vi "Main.vi"() -> ()   [LabVIEW 2020]
uses:
  <vilib>/SAPHIR/ViBox - XControls/XTab/XTab.xctl
  Global.vi
panel:
  out "名称":string="C-EPS生产质量追溯系统"
  in  "XTab":refnum<vi>(xcontrol)
  out "时间：":string
  out "权限：":string
  out "用户：":string
  # "广东和氏工业技术集团股份有限公司"
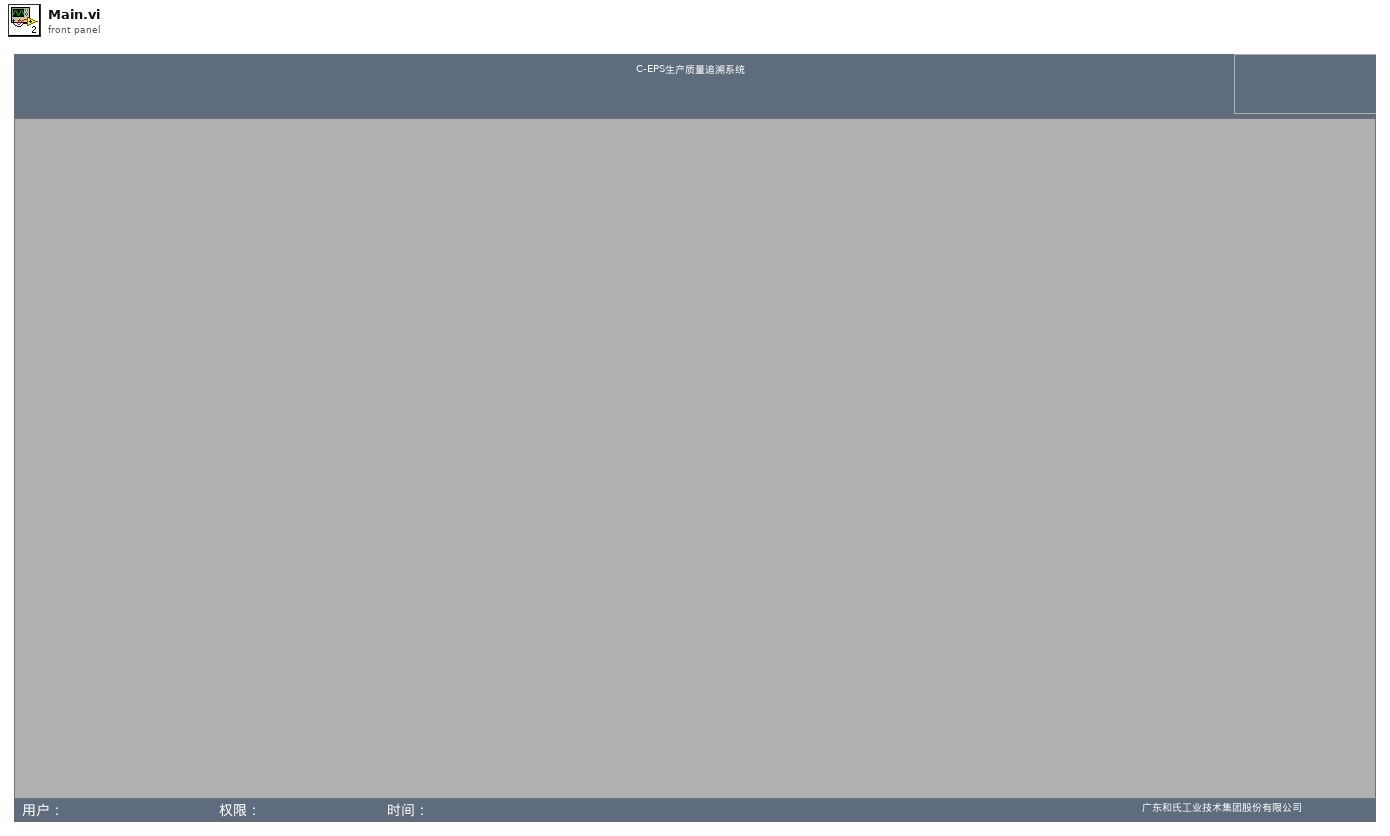
[diagram p1: front panel]
types:
  T1 = enum32{"Invalid", "Standard", "Closed", "Hidden", "Minimized", "Maximized"}
  T2 = cluster{"用户编号":string, "用户名":string, "用户密码(密文)":string, "用户权限":string}
  T3 = enum32{"invalid app kind", "Development System", "Run Time System", "Student Edition", "Embedded LabVIEW", "Evaluation", "Custom"}
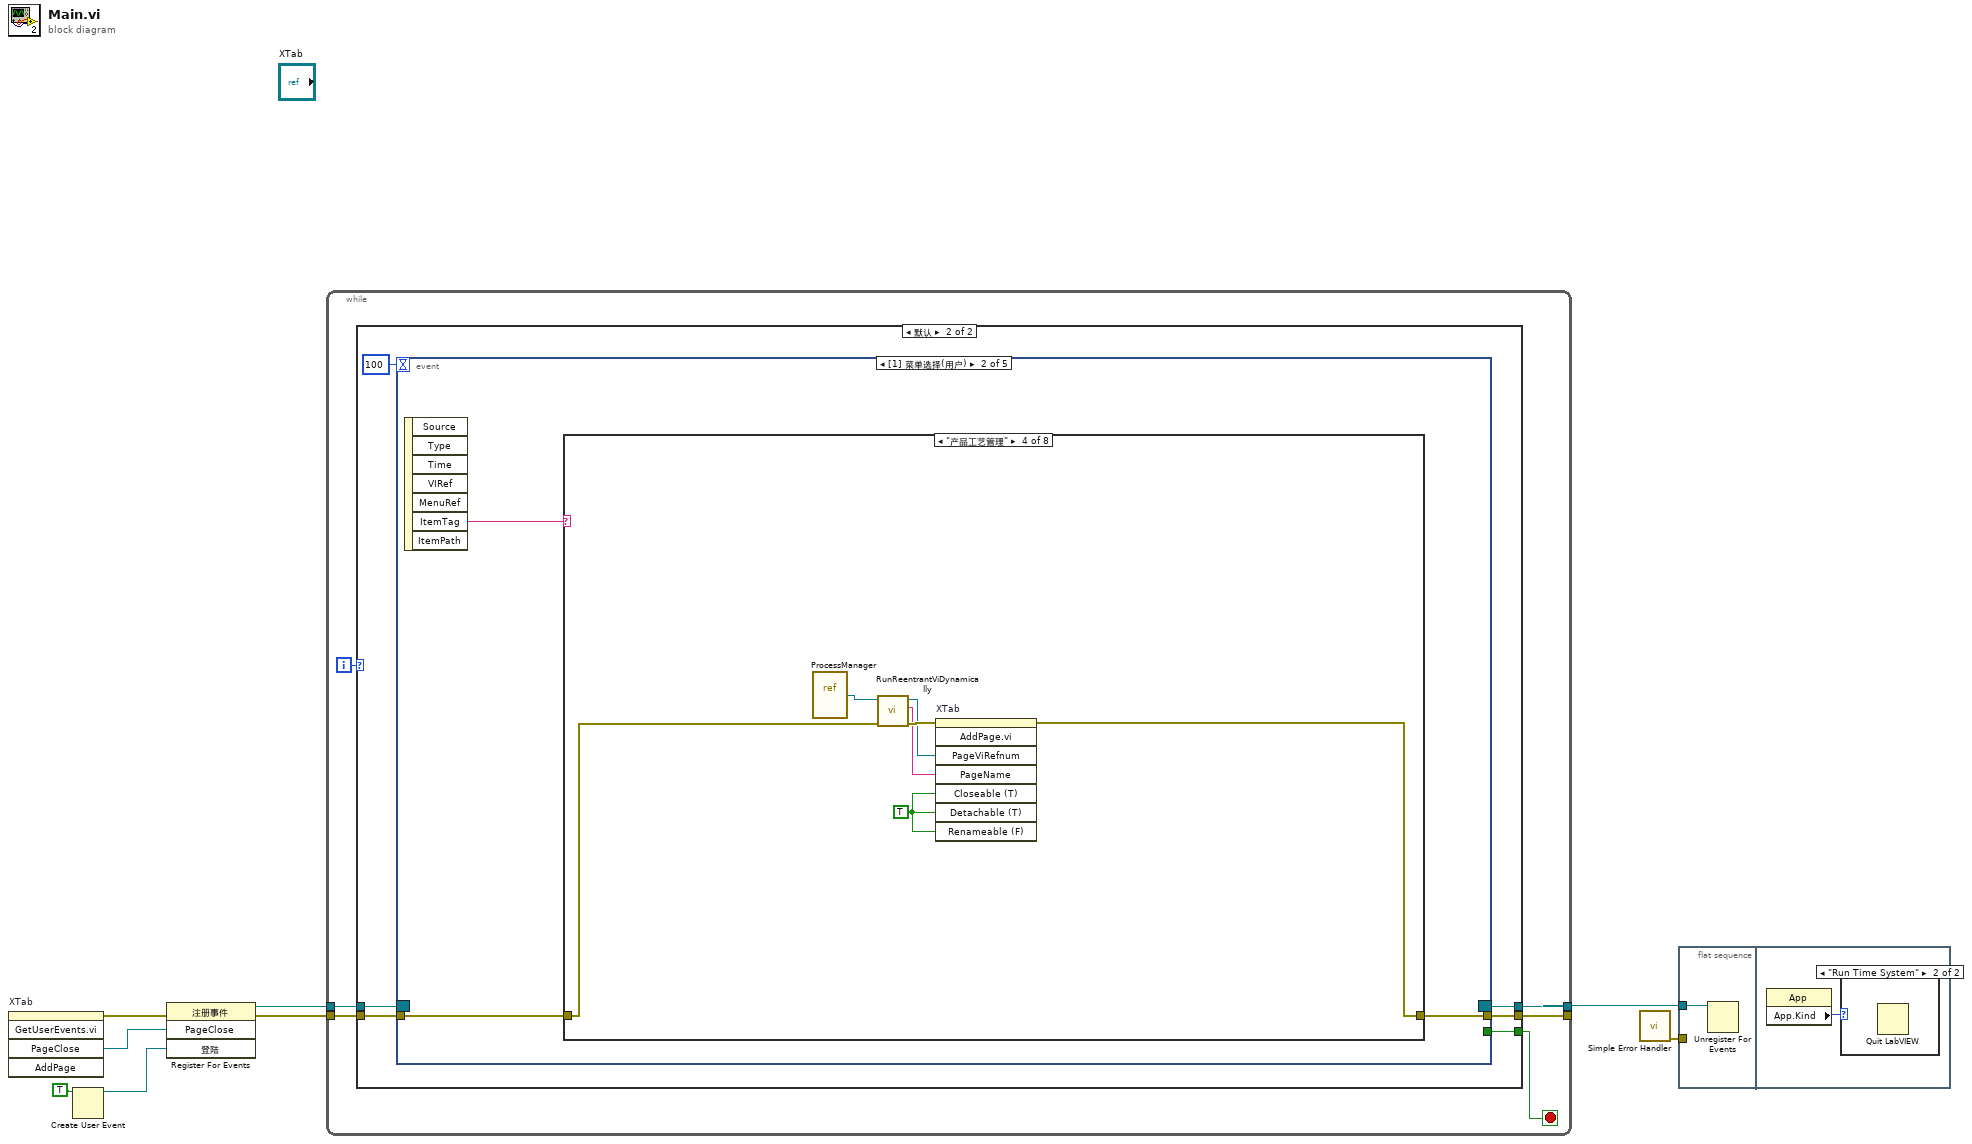
[diagram p0: block diagram]
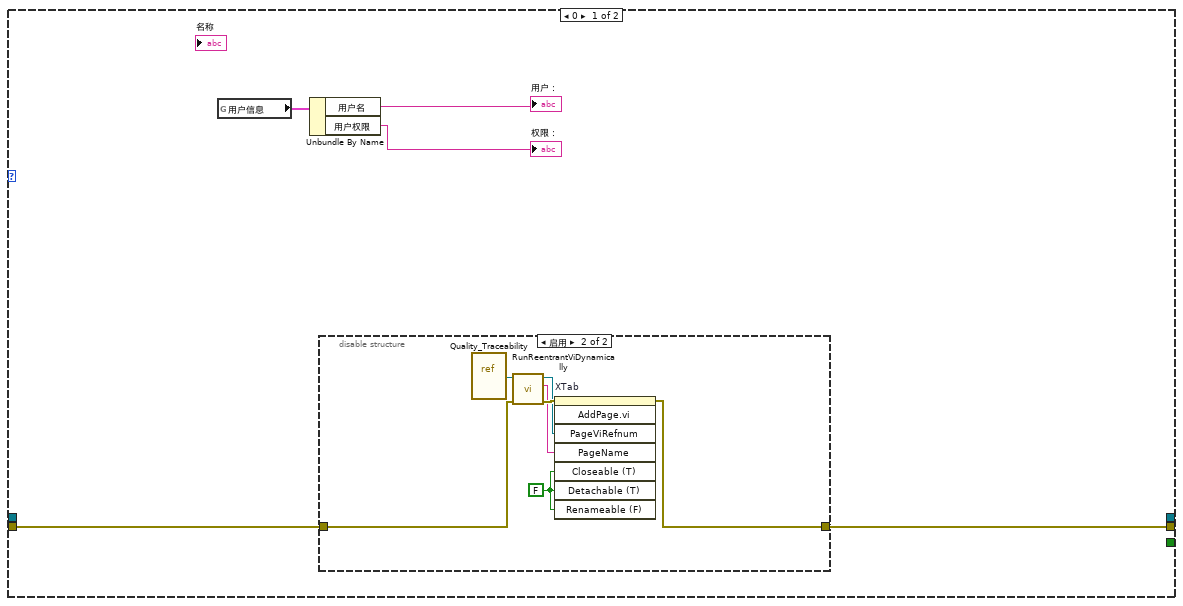
[diagram p3: hidden frame]
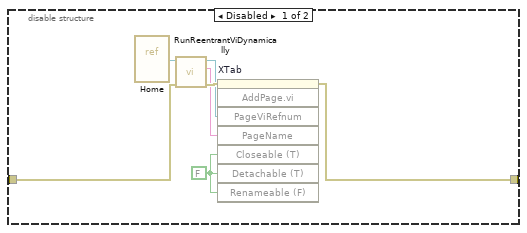
[diagram p4: hidden frame]
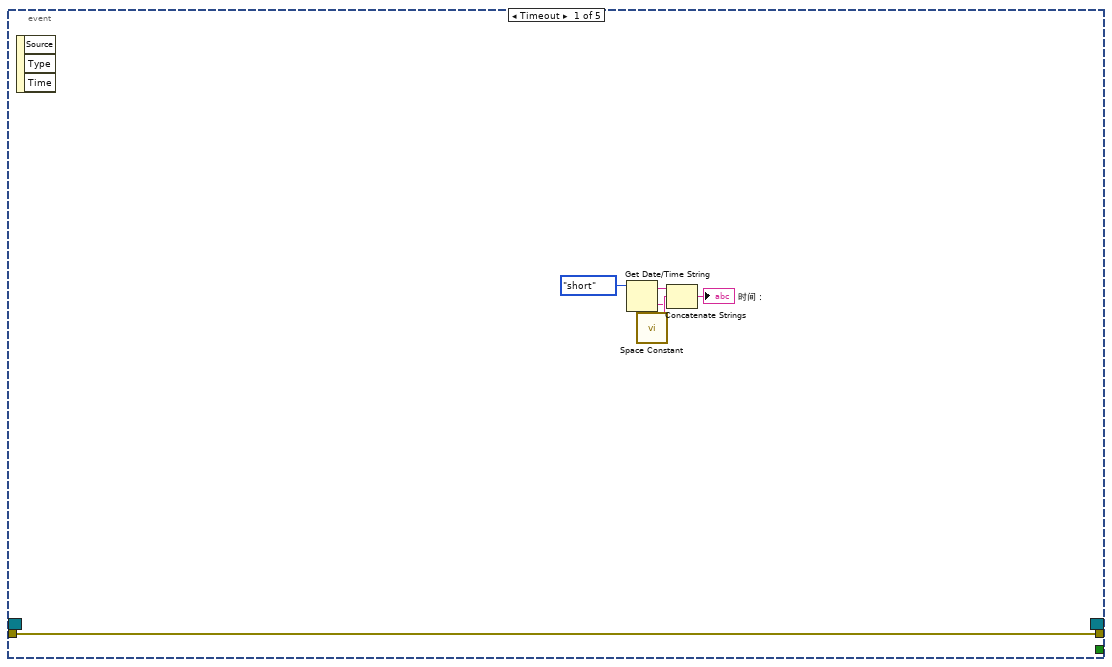
[diagram p5: hidden frame]
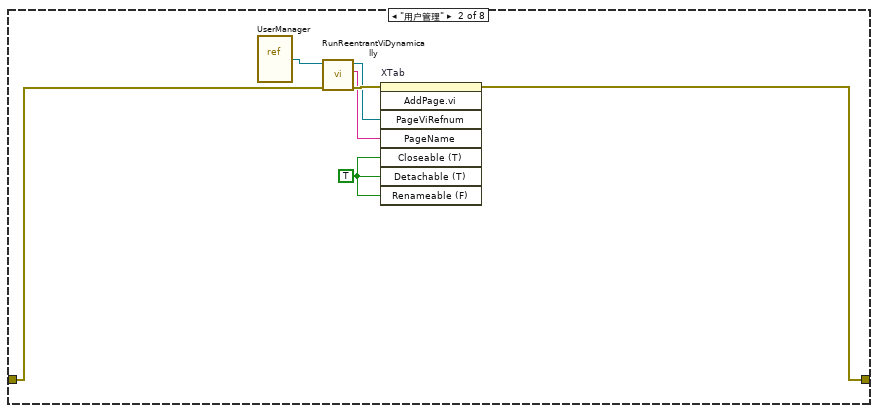
[diagram p7: hidden frame]
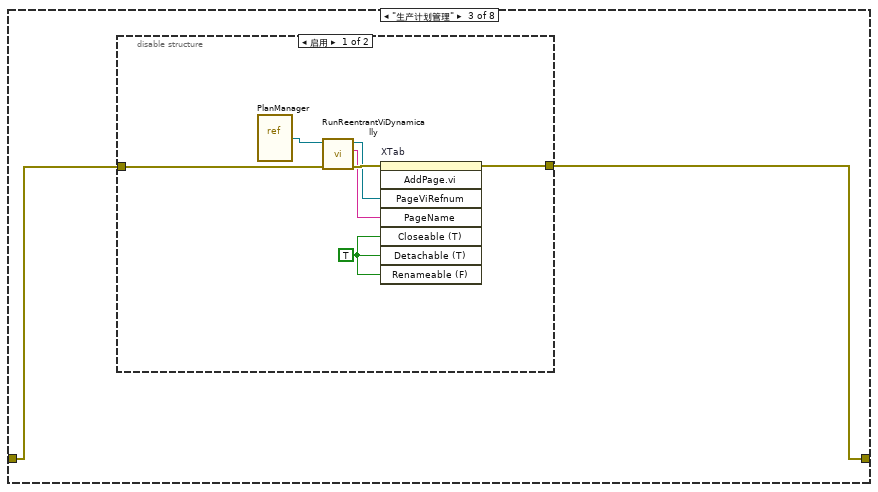
[diagram p8: hidden frame]
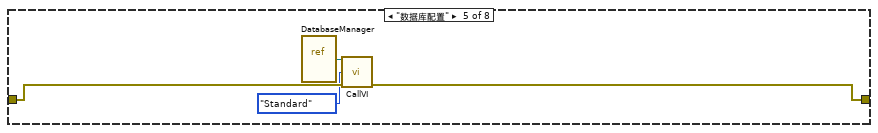
[diagram p10: hidden frame]
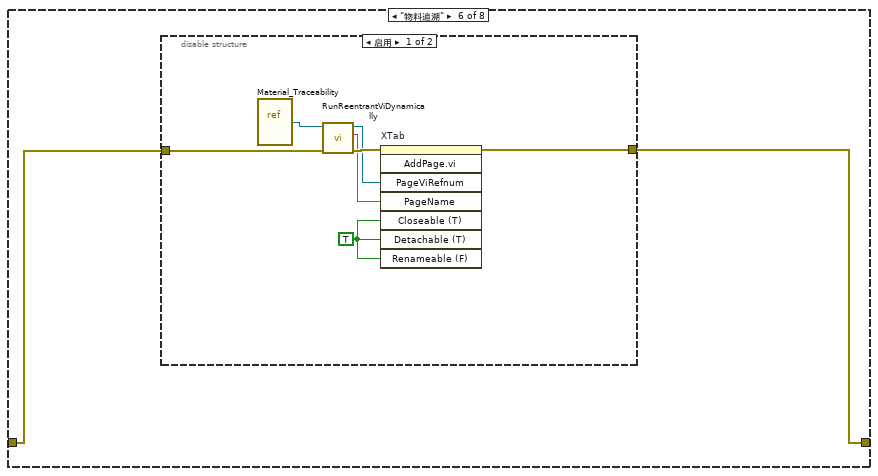
[diagram p11: hidden frame]
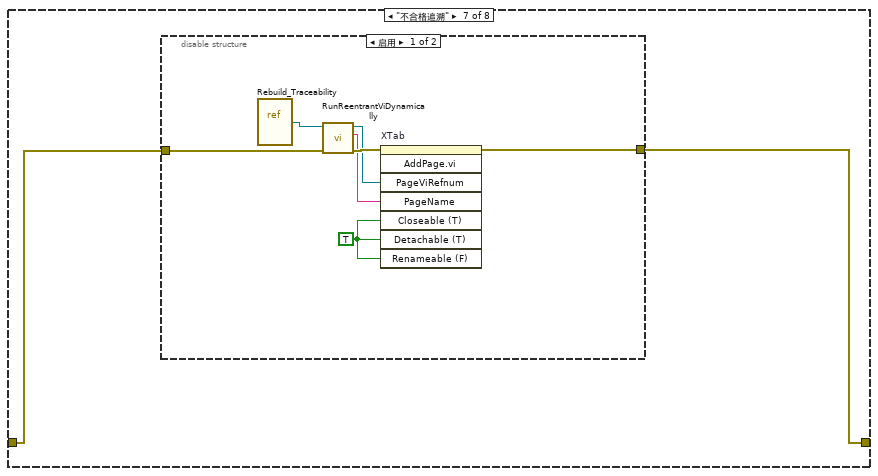
[diagram p13: hidden frame]
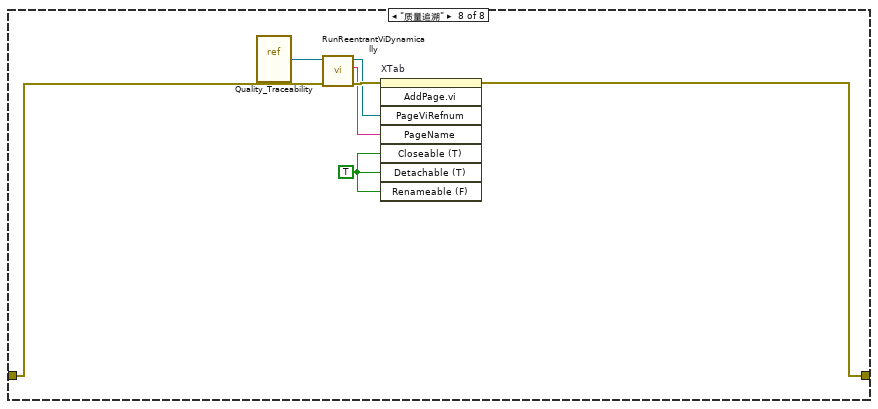
[diagram p15: hidden frame]
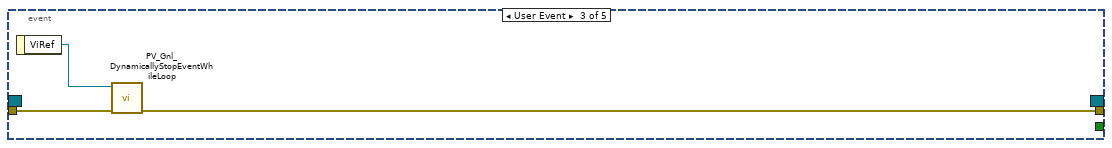
[diagram p16: hidden frame]
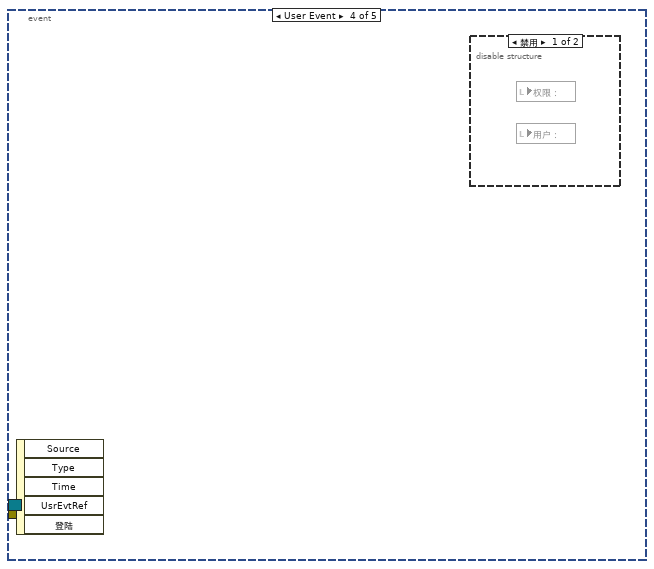
[diagram p17: hidden frame]
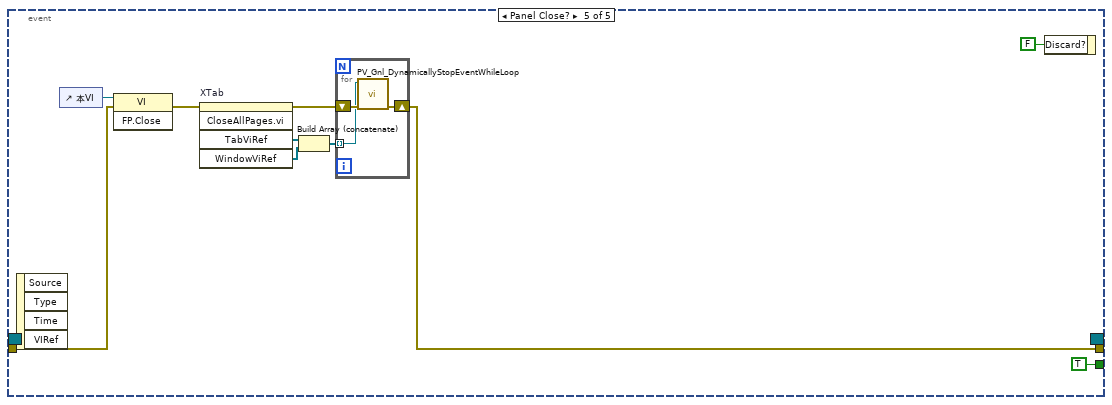
[diagram p19: hidden frame]
diagram:
  n1 = invoke on="XTab" class="XTab (严格)" method="GetUserEvents.vi"() -> (error out=w3:errorcluster, "PageClose"=w8:refnum<user-event>)  [unwired: 5 in, 3 out]
  n2 = Create User Event(user event datatype=TRUE ("登陆")) -> (user event=w1:refnum<user-event>)  [unwired: 1 in, 1 out]
  n3 = register-events(error in=w3, w8, w1) -> (reference out=w6:refnum<event-registration>, error out=w4:errorcluster)  [unwired: 1 in]
  n4 = while {
    tunnel: w6 -> [w13]
    tunnel: [w12] -> w5
    tunnel: w4 -> [w11]
    tunnel: [w10] -> _
    i -> [w14]
    stop <- w9 stop-if-true
    n5 = case shown="默认" w14 {
      tunnel: w13 -> [_ w39]
      tunnel: [_ w38] -> w12
      tunnel: w11 -> [w19 w37]
      tunnel: [w18 w36] -> w10
      tunnel: [_ w35] -> w9
      frame 0 {
        n6 = global read "Global.vi" "用户信息"() -> (w17:T2)
        n7 = Unbundle By Name(w17) -> ("用户名"=→"用户：":string, "用户权限"=→"权限：":string)
        n8 = disable-structure shown="启用" {
          disable-tunnel: w19 -> [w21 w28]
          disable-tunnel: [w20 w27] -> w18
          frame Disabled {
            w26 = FALSE ("Closeable (T)")
            n9 = vi-ref "Home.vi"() -> (w25:refnum<vi>)
            n10 = call "RunReentrantViDynamically.vi"("error in"=w21, "ViRefIn"=w25) -> ("error out"=w24:errorcluster, "VIName"=w23:string, "ViRefNum"=w22:refnum<vi>)  [unwired: 7 in]
            n11 = invoke on="XTab" class="XTab (严格)" method="AddPage.vi"(error in=w24, "PageViRefnum"=w22, "PageName"=w23, "Closeable (T)"=w26, "Detachable (T)"=w26, "Renameable (F)"=w26) -> (error out=w20:errorcluster)  [unwired: 2 in, 7 out]
          }
          frame Enabled {
            w29 = FALSE ("Closeable (T)")
            n12 = vi-ref "Quality_Traceability.vi"() -> (w33:refnum<vi>)
            n13 = call "RunReentrantViDynamically.vi"("error in"=w28, "ViRefIn"=w33) -> ("error out"=w32:errorcluster, "VIName"=w31:string, "ViRefNum"=w30:refnum<vi>)  [unwired: 7 in]
            n14 = invoke on="XTab" class="XTab (严格)" method="AddPage.vi"(error in=w32, "PageViRefnum"=w30, "PageName"=w31, "Closeable (T)"=w29, "Detachable (T)"=w29, "Renameable (F)"=w29) -> (error out=w27:errorcluster)  [unwired: 2 in, 7 out]
          }
        }
      }
      frame Default {
        n15 = event shown="[1] 菜单选择(用户)" {
          selector: w39 -> [_ _ _ _ _]
          dyn-events: [_ _ _ _ _] -> w38
          timeout: 100 -> [_ _ _ _ _]
          tunnel: w37 -> [w45 w47 w107 _ w109]
          tunnel: [w45 w46 w106 _ w114] -> w36
          tunnel: [_ _ _ _ TRUE] -> w35
          event Timeout {
            n16 = event-data() -> ()  [unwired: 1 in, 3 out]
            n17 = Get Date/Time String(date format (0)=enum16{"short", "long", "abbreviated"}."short" ("日期格式(0)")) -> (date string=w41:string, time string=w43:string)  [unwired: 2 in]
            n18 = call <vilib>:"Space Constant.vi"() -> ("String"=w44:string)
            n19 = Concatenate Strings(w41, w44, w43) -> (→"时间：":string)
          }
          event Menu Selection (User) {
            n20 = event-data() -> ("ItemTag"=w48:string)  [unwired: 1 in, 6 out]
            n21 = case shown="\"产品工艺管理\"" w48 {
              tunnel: w47 -> [w49 w52 w58 w73 w76 w79 w89 w100]
              tunnel: [w49 w51 w57 w72 w75 w78 w88 w99] -> w46
              frame Default {
              }
              frame "用户管理" {
                w56 = TRUE ("Closeable (T)")
                n22 = vi-ref "UserManager.vi"() -> (w50:refnum<vi>)
                n23 = call "RunReentrantViDynamically.vi"("error in"=w52, "ViRefIn"=w50) -> ("error out"=w55:errorcluster, "VIName"=w54:string, "ViRefNum"=w53:refnum<vi>)  [unwired: 7 in]
                n24 = invoke on="XTab" class="XTab (严格)" method="AddPage.vi"(error in=w55, "PageViRefnum"=w53, "PageName"=w54, "Closeable (T)"=w56, "Detachable (T)"=w56, "Renameable (F)"=w56) -> (error out=w51:errorcluster)  [unwired: 2 in, 7 out]
              }
              frame "生产计划管理" {
                n25 = disable-structure shown="启用" {
                  disable-tunnel: w58 -> [w61 w66]
                  disable-tunnel: [w60 w66] -> w57
                  frame Enabled {
                    w65 = TRUE ("Closeable (T)")
                    n26 = vi-ref "PlanManager.vi"() -> (w59:refnum<vi>)
                    n27 = call "RunReentrantViDynamically.vi"("error in"=w61, "ViRefIn"=w59) -> ("error out"=w64:errorcluster, "VIName"=w63:string, "ViRefNum"=w62:refnum<vi>)  [unwired: 7 in]
                    n28 = invoke on="XTab" class="XTab (严格)" method="AddPage.vi"(error in=w64, "PageViRefnum"=w62, "PageName"=w63, "Closeable (T)"=w65, "Detachable (T)"=w65, "Renameable (F)"=w65) -> (error out=w60:errorcluster)  [unwired: 2 in, 7 out]
                  }
                  frame Disabled {
                  }
                }
              }
              frame "产品工艺管理" {
                w71 = TRUE ("Closeable (T)")
                n29 = vi-ref "ProcessManager.vi"() -> (w67:refnum<vi>)
                n30 = call "RunReentrantViDynamically.vi"("error in"=w73, "ViRefIn"=w67) -> ("error out"=w70:errorcluster, "VIName"=w69:string, "ViRefNum"=w68:refnum<vi>)  [unwired: 7 in]
                n31 = invoke on="XTab" class="XTab (严格)" method="AddPage.vi"(error in=w70, "PageViRefnum"=w68, "PageName"=w69, "Closeable (T)"=w71, "Detachable (T)"=w71, "Renameable (F)"=w71) -> (error out=w72:errorcluster)  [unwired: 2 in, 7 out]
              }
              frame "数据库配置" {
                n32 = vi-ref "DatabaseManager.vi"() -> (w77:refnum<vi>)
                n33 = call "CallVI.vi"("VI引用"=w77, "状态"=T1."Standard", "错误输入"=w76) -> ("错误输出"=w75:errorcluster)  [unwired: 10 in, 2 out]
              }
              frame "物料追溯" {
                n34 = disable-structure shown="启用" {
                  disable-tunnel: w79 -> [w82 w87]
                  disable-tunnel: [w81 w87] -> w78
                  frame Enabled {
                    w86 = TRUE ("Closeable (T)")
                    n35 = vi-ref "Material_Traceability.vi"() -> (w80:refnum<vi>)
                    n36 = call "RunReentrantViDynamically.vi"("error in"=w82, "ViRefIn"=w80) -> ("error out"=w85:errorcluster, "VIName"=w84:string, "ViRefNum"=w83:refnum<vi>)  [unwired: 7 in]
                    n37 = invoke on="XTab" class="XTab (严格)" method="AddPage.vi"(error in=w85, "PageViRefnum"=w83, "PageName"=w84, "Closeable (T)"=w86, "Detachable (T)"=w86, "Renameable (F)"=w86) -> (error out=w81:errorcluster)  [unwired: 2 in, 7 out]
                  }
                  frame Disabled {
                  }
                }
              }
              frame "不合格追溯" {
                n38 = disable-structure shown="启用" {
                  disable-tunnel: w89 -> [w92 w97]
                  disable-tunnel: [w91 w97] -> w88
                  frame Enabled {
                    w96 = TRUE ("Closeable (T)")
                    n39 = vi-ref "Rebuild_Traceability.vi"() -> (w90:refnum<vi>)
                    n40 = call "RunReentrantViDynamically.vi"("error in"=w92, "ViRefIn"=w90) -> ("error out"=w95:errorcluster, "VIName"=w94:string, "ViRefNum"=w93:refnum<vi>)  [unwired: 7 in]
                    n41 = invoke on="XTab" class="XTab (严格)" method="AddPage.vi"(error in=w95, "PageViRefnum"=w93, "PageName"=w94, "Closeable (T)"=w96, "Detachable (T)"=w96, "Renameable (F)"=w96) -> (error out=w91:errorcluster)  [unwired: 2 in, 7 out]
                  }
                  frame Disabled {
                  }
                }
              }
              frame "质量追溯" {
                w104 = TRUE ("Closeable (T)")
                n42 = vi-ref "Quality_Traceability.vi"() -> (w98:refnum<vi>)
                n43 = call "RunReentrantViDynamically.vi"("error in"=w100, "ViRefIn"=w98) -> ("error out"=w103:errorcluster, "VIName"=w102:string, "ViRefNum"=w101:refnum<vi>)  [unwired: 7 in]
                n44 = invoke on="XTab" class="XTab (严格)" method="AddPage.vi"(error in=w103, "PageViRefnum"=w101, "PageName"=w102, "Closeable (T)"=w104, "Detachable (T)"=w104, "Renameable (F)"=w104) -> (error out=w99:errorcluster)  [unwired: 2 in, 7 out]
              }
            }
          }
          event User Event {
            n45 = event-data() -> ("ViRef"=w105:refnum<vi>)  [unwired: 1 in]
            n46 = call "PV_Gnl_DynamicallyStopEventWhileLoop.vi"("error in"=w107, "ViRefNum"=w105) -> ("error out"=w106:errorcluster)  [unwired: 8 in, 1 out]
          }
          event User Event {
            n47 = event-data() -> ()  [unwired: 1 in, 5 out]
            n48 = disable-structure shown="禁用" {
              frame Disabled {
                n49 = local read "权限："() -> ()  [unwired: 1 in]
                n50 = local read "用户："() -> ()  [unwired: 1 in]
              }
              frame Enabled {
              }
            }
          }
          event Panel Close? {
            n51 = event-data() -> ()  [unwired: 1 in, 4 out]
            n52 = control-ref of="本VI"() -> (w110:refnum<vi>)
            n53 = invoke class="VI" method="FP.Close"(reference=w110, error in=w109) -> (error out=w108:errorcluster)  [unwired: 1 in, 2 out]
            n54 = invoke on="XTab" class="XTab (严格)" method="CloseAllPages.vi"(error in=w108) -> (error out=w115:errorcluster, "TabViRef"=w117:refnum<vi>[], "WindowViRef"=w116:refnum<vi>[])  [unwired: 4 in, 2 out]
            n55 = Build Array (concatenate)(w117, w116) -> (w113:refnum<vi>[])
            n56 = for {
              tunnel: w113 -> [w118] mode=indexing
              shift-right: [w119] -> w114
              shift-left: w115 -> [w120]
              n57 = call "PV_Gnl_DynamicallyStopEventWhileLoop.vi"("error in"=w120, "ViRefNum"=w118) -> ("error out"=w119:errorcluster)  [unwired: 8 in, 1 out]
            }
            n58 = event-data("Discard?"=FALSE ("放弃？")) -> ()  [unwired: 1 in, 1 out]
          }
        }
      }
    }
  }
  n59 = call <vilib>:"Simple Error Handler.vi"() -> ("error out"=w7:errorcluster)  [unwired: 2 in, 7 out]
  n60 = flat-sequence {
    tunnel: w7 -> [_]
    tunnel: w5 -> [w121]
    frame #0 {
      n61 = Unregister For Events(event registration refnum=w121) -> ()  [unwired: 1 in, 1 out]
    }
    frame #1 {
      n62 = property class="App"() -> ("App.Kind"=w122:T3)  [unwired: 2 in, 2 out]
      n63 = case shown="\"Run Time System\"" w122 {
        frame Default {
        }
        frame "Run Time System" {
          n64 = Quit LabVIEW() -> ()  [unwired: 1 out]
        }
      }
    }
  }
